vi "to string array.vi"(8 "error in (no error)":errorcluster, 11 "module configuration in":refnum<class "TBM module configuration.lvclass">) -> (0 "error out":errorcluster, 1 "Array":string[][](array[string]), 2 "version":string, 3 "module configuration out":refnum<class "TBM module configuration.lvclass">)   [LabVIEW 2014, in "TBM module configuration.lvclass"]
uses:
  TBM module configuration.lvclass
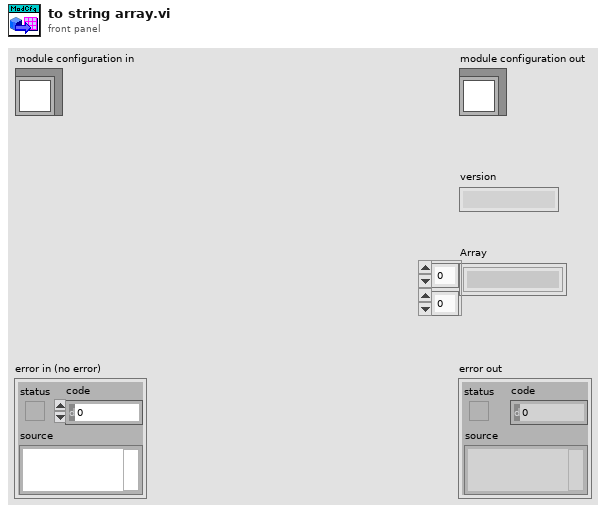
[diagram p1: front panel]
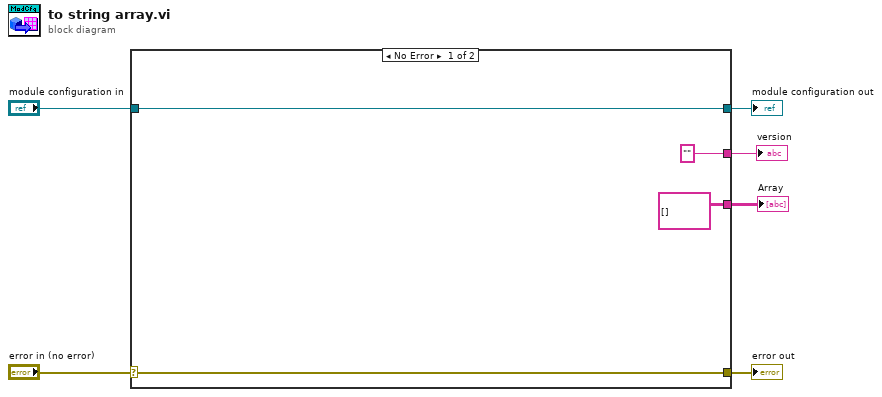
[diagram p0: block diagram]
diagram:
  n1 = case shown="No Error" "error in (no error)" {
    selector: "error in (no error)" -> [w9 w12]
    tunnel: [w9 w12] -> w5
    tunnel: [w10 w11] -> w3
    tunnel: "module configuration in" -> [w10 w11]
    tunnel: [string[][] [] ("Array") _] -> w2
    tunnel: ["" ("version") _] -> w1
    frame No Error {
    }
    frame Error {
    }
  }
  "error out" <- w5
  "module configuration out" <- w3
  "Array" <- w2
  "version" <- w1
